vi "Main_Old.vi"() -> ()   [LabVIEW 2018]
uses:
  classes/Tushars Events Toolkit/Software/Modules/EventClient_ObjectReference.ctl
  classes/Variable Manager/VariableManager_Bool.vi
  Strict Type Controls/Settings Operation.ctl
  classes/Variable Manager/VariableManager_Double.vi
  <vilib>/Utility/file.llb/Write To Spreadsheet File (string).vi
panel:
  out "Quit":bool
  out "error out":errorcluster
  in  "error in (no error)":errorcluster
  in  "abort":bool
  in  "start":bool
  out "Test Status":bool
  out "statusMerlin":bool
  out "statusMC":bool
  out "statusPS":bool
  out "statusSM":bool
  in  "Start Merlin":bool
  in  "Start Monochromator":bool
  in  "Start Power Supply":bool
  in  "Start Source Meter":bool
  out "Value":dbl format="%#.7f mV"
  out "Measuring":dbl format="%#.7f nm"
  out "Voltage":dbl format="%#.7f mV"
  in  "tab":T1(tab)
  in  "Path For VT":path
  in  "exportVT":bool
  out "VTGraph":cluster{dbl[], dbl[]}(graph)
  in  "Test Mode":enum16{"Time Mode", "dV/dt Mode"}(ring)
  in  "Log Interval":u32=50 min=100 step=1 format="%.0f mSec"
  in  "Test Time":dbl step=1.0 format="%<%H:%M:%S>t"
  out "Time Remaining":dbl format="%<%H:%M:%S>t"
  in  "Target dV/dt":dbl format="%#.9f mV"
  in  "Lock In time":dbl step=1.0 format="%<%H:%M:%S>t"
  out "dV/dt":dbl format="%#.11f mV"
  out "Locked Time":dbl step=1.0 format="%<%H:%M:%S>t"
  in  "Perform Test After":T1(ring)=enum."Voltage Vs Wavelength"
  out "gratSetup?":bool
  in  "portD":bool
  in  "portA":bool
  in  "Path For Sweep":path
  in  "exportSweep":bool
  out "sweep":cluster{dbl[], dbl[]}[](graph)
  in  "Settling Time (ms)":dbl=5000.0
  in  "To":dbl=1000.0
  in  "Step":dbl=100.0
  in  "From":dbl=100.0
  in  "SetSlit":bool
  in  "SetGrating":bool
  in  "SetMonochromator":bool
  in  "Wavelength":dbl
  in  "Slit":string(combo)
  in  "GratingNo":u8=1 min=1 max=3 step=1
  in  "set Lock in":bool
  in  "#Stages":enum16{"None", "1 Pole", "2 Pole"}(ring)
  in  "Phase":enum16{"1 Phase", "2 Phase"}(ring)
  in  "SyncMode":T2(ring)
  in  "Time Const":T3(ring)
  in  "Sweep Results":i32(listbox)
  out "DCCurrent":dbl format="%#.4f A"
  out "DCVoltage":dbl format="%#.4f V"
  in  "Command":T4(ring)
  in  "Parm 4":dbl format="%#.6f"
  in  "Parm 3":dbl format="%#.6f"
  in  "openScript":bool
  in  "exportScript":bool
  in  "Path For Script":path
  in  "update":bool
  out "scriptGraph":cluster{dbl[], dbl[]}(graph)
  in  "Parm 2":dbl format="%#.6f"
  in  "Parm 1":dbl format="%#.6f"
  in  "script":i32(listbox)
  in  "add":bool
  in  "remove":bool
  in  "exportScriptResults":bool
  in  "Path For Script Results":path
  in  "Script Avg Interval":u32=50 min=100 step=1 format="%.0f mSec"
  # "Status"
  # "Test Type"
  # "Test Time"
  # "Voltage Results"
  # "Monochromator"
  # "Lock In Amplifier"
  # "Sweep"
  # "Merlin"
  # "NOTE:\n1. if this LED is OFF then GPIB is not connected...\n2. Close program before power off Instruments..."
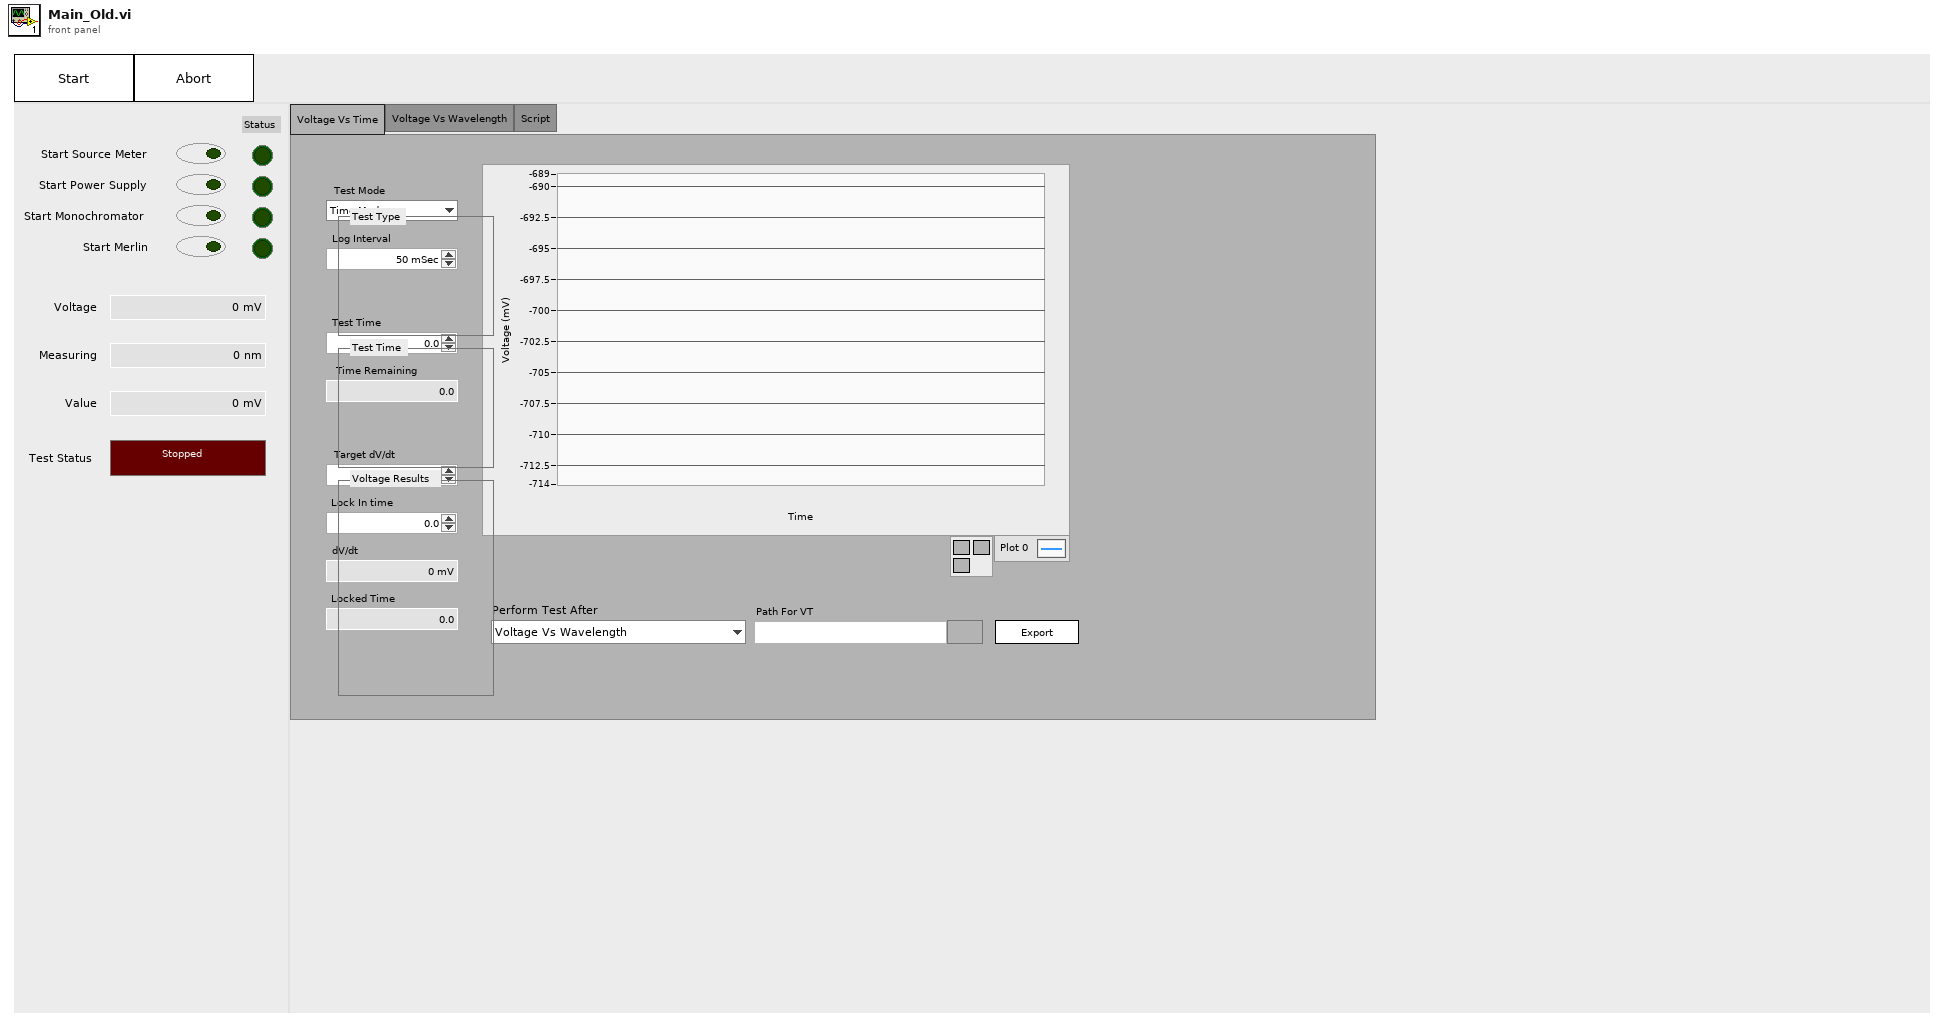
[diagram p1: front panel]
types:
  T1 = enum32{"Voltage Vs Time", "Voltage Vs Wavelength", "Script"}
  T2 = enum16{"Int Chop Off", "Int Chop On", "Ext Chop Off", "Ext Chop On"}
  T3 = enum16{".003s", ".010s", ".030s", ".100s", ".300s", "1.00s", "3.00s", "10.0s", "30.0s", "100s"}
  T4 = enum16{"selectChannel", "setDCVoltage", "setDCCurrent", "setVoltageSteps", "wait"}
  T5 = cluster{"startTime":u32, "lastUpdate":u32, "lastVoltage":dbl, "run?":bool, "From":dbl, "time":dbl[], "MerlinVal":dbl[], "SMVolt":dbl[], "sweepType":enum16{"ASC", "DESC"}, "Wavlnth":dbl[], "Test Mode":enum16{"Time Mode", "dV/dt Mode"}, "tab":enum32{"Voltage Vs Time", "Voltage Vs Wavelength", "Script"}, "script":string[][], "dV/dt":dbl[], "graphUpdate":u32}
  T6 = typedef "EventClient_ObjectReference.ctl" = refnum<k1>
  T7 = typedef "Settings Operation.ctl" = enum8{"Get Value", "Set Value", "Read File", "Write File", "Write Stored Value"}
  T8 = cluster{"GratingNo":u8, "Slit":string, "wavelength":dbl}
  T9 = cluster{"#Stages":enum16{"None", "1 Pole", "2 Pole"}, "Phase":enum16{"1 Phase", "2 Phase"}, "SyncMode":enum16{"Int Chop Off", "Int Chop On", "Ext Chop Off", "Ext Chop On"}, "Time Const":enum16{".003s", ".010s", ".030s", ".100s", ".300s", "1.00s", "3.00s", "10.0s", "30.0s", "100s"}}
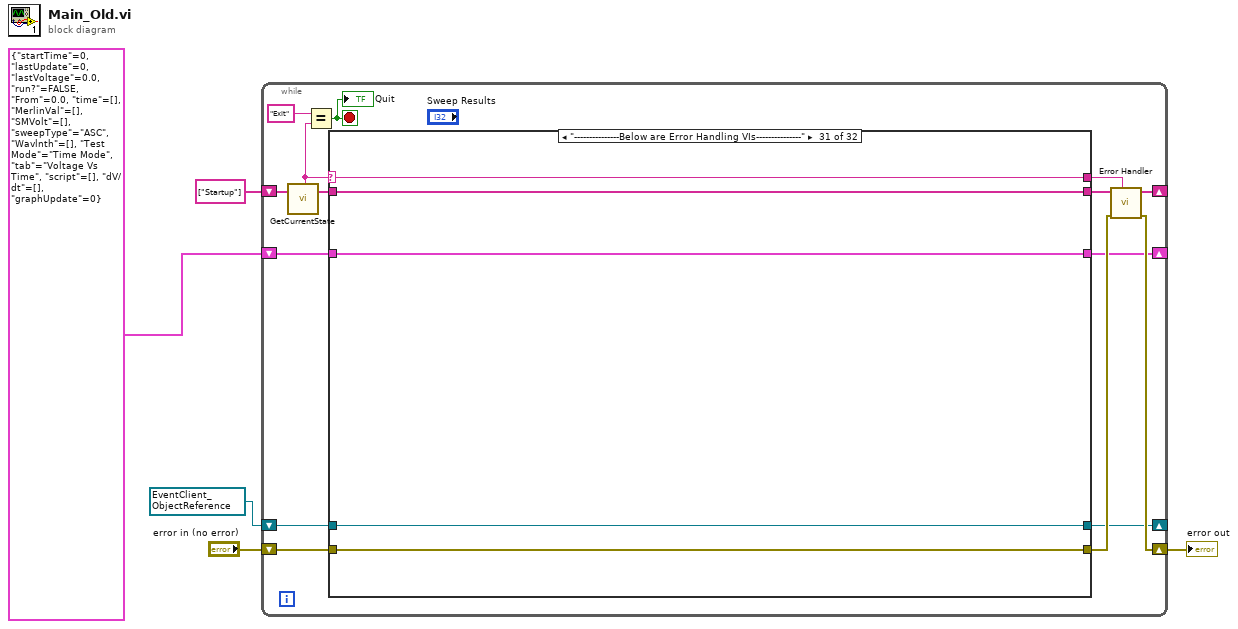
[diagram p0: block diagram]
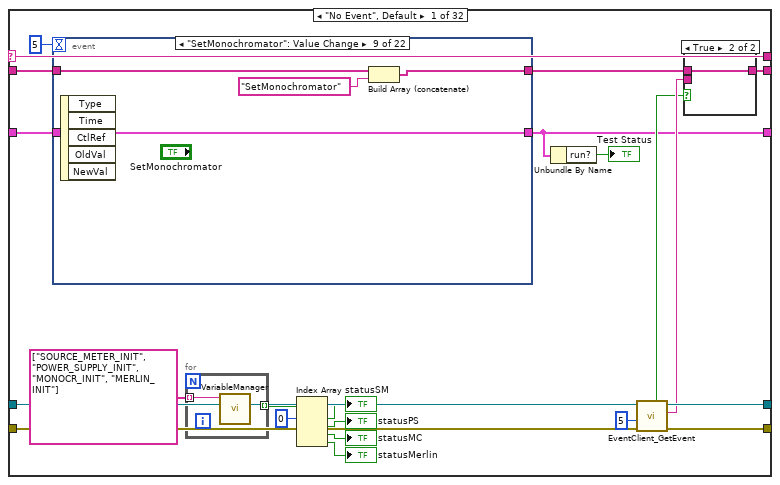
[diagram p2: hidden frame]
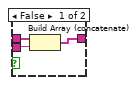
[diagram p3: hidden frame]
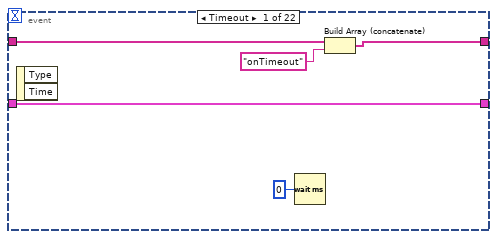
[diagram p4: hidden frame]
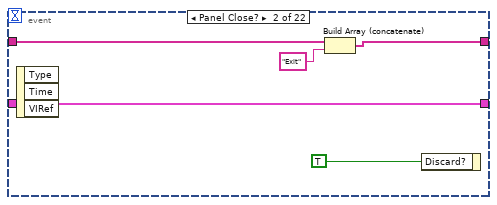
[diagram p5: hidden frame]
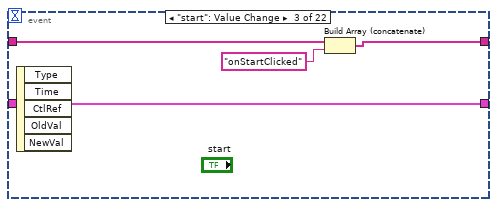
[diagram p6: hidden frame]
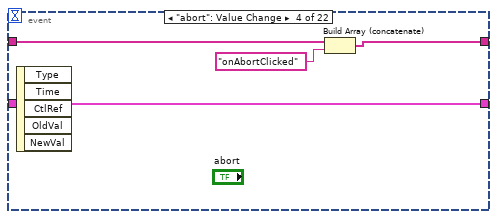
[diagram p7: hidden frame]
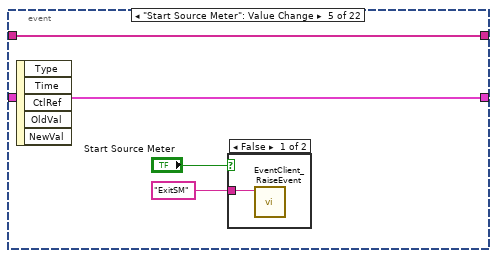
[diagram p8: hidden frame]
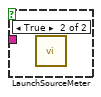
[diagram p9: hidden frame]
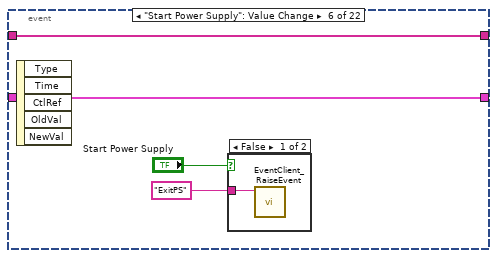
[diagram p10: hidden frame]
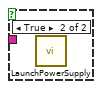
[diagram p11: hidden frame]
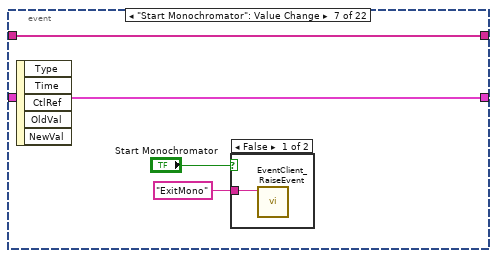
[diagram p12: hidden frame]
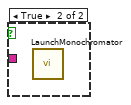
[diagram p13: hidden frame]
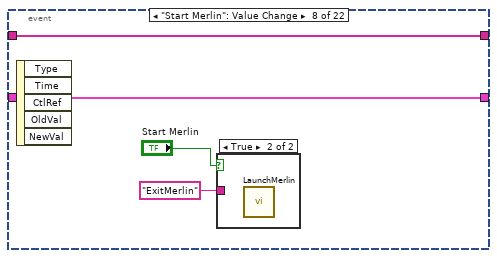
[diagram p14: hidden frame]
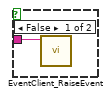
[diagram p15: hidden frame]
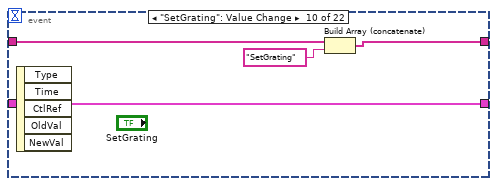
[diagram p16: hidden frame]
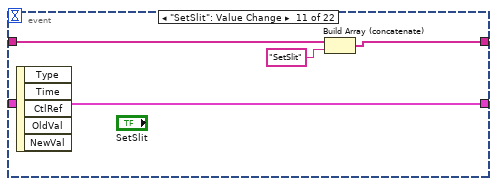
[diagram p17: hidden frame]
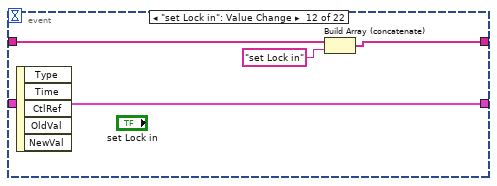
[diagram p18: hidden frame]
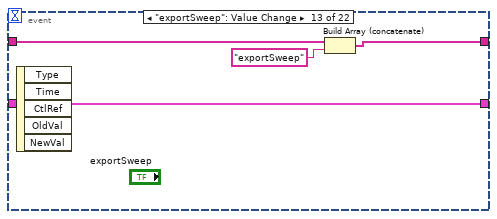
[diagram p19: hidden frame]
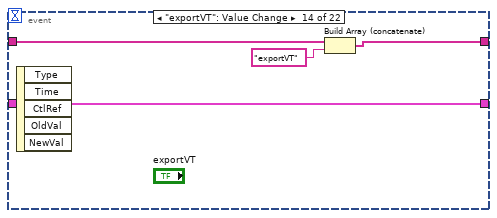
[diagram p20: hidden frame]
diagram:
  w2 = T6 refnum items=["EventClient"] ("reference")
  n1 = while {
    shift-right: [w16] -> _
    shift-left: string[] ["Startup"] ("State Array Out") -> [w20]
    shift-right: [w12] -> w3
    shift-left: "error in (no error)" -> [w13]
    shift-right: [w9] -> _
    shift-left: w2 -> [w8]
    shift-right: [w6] -> _
    shift-left: T5 {"startTime"=0, "lastUpdate"=0, "lastVoltage"=0.0, "run?"=FALSE, "From"=0.0, "time"=[], "MerlinVal"=[], "SMVolt"=[], "sweepType"=enum."ASC", "Wavlnth"=[], "Test Mode"=enum."Time Mode", "tab"=enum."Voltage Vs Time", "script"=[], "dV/dt"=[], "graphUpdate"=0} -> [w7]
    stop <- w17 stop-if-true
    n2 = call "GetCurrentState.vi"("State Array In"=w20) -> ("Current State"=w10:string, "State Array Out"=w19:string[])  [unwired: 17 in]
    n3 = Equal?(x="Exit", y=w10) -> (x = y?=w17:bool)
    "Quit" <- w17
    n4 = case shown="\"---------------Below are Error Handling VIs---------------\"" w10 {
      selector: w10 -> [w42 w172 w174 w184 w198 w208 w225 w242 w250 w258 w266 w290 w305 w315 w330 w348 w356 w367 w374 w386 w394 w404 w415 w420 w456 w496 w553 w577 w591 w655 w678 w694]
      tunnel: w19 -> [w41 w171 w180 w185 w199 w209 w226 w243 w251 w259 w267 w291 w306 w316 w331 w349 w364 w371 w378 w390 w395 w405 w416 w421 w457 w484 w554 w578 w582 w656 w677 w681]
      tunnel: [w32 w170 w180 w185 w199 w209 w226 w243 w251 w259 w267 w291 w306 w316 w331 w349 w364 w371 w378 w390 w395 w405 w416 w421 w457 w483 w554 w578 w583 w656 w677 w681] -> w15
      tunnel: [w37 w164 w175 w183 w197 w207 w224 w241 w249 w252 w260 w289 w304 w314 w329 w347 w357 w368 w375 w387 w393 w400 w411 w419 w450 w495 w552 w576 w590 w631 w676 errorcluster {"status"=FALSE, "code"=0, "source"=""} ("error in (no error)")] -> w11
      tunnel: [w42 w172 w174 w184 w198 w208 w225 w242 w250 w258 w266 w290 w305 w315 w330 w348 w356 w367 w374 w386 w394 w404 w415 w420 w456 w496 w553 w577 w591 w655 w678 w694] -> w14
      tunnel: w13 -> [w38 w159 w178 w183 w197 w207 w224 w241 w249 w253 w261 w289 w304 w314 w329 w347 w358 w369 w376 w388 w393 w402 w413 w419 w451 w495 w552 w576 w590 w632 w676 w682]
      tunnel: [w36 w162 w177 w182 w196 w206 w223 w240 w248 w257 w265 w288 w303 w313 w328 w346 w363 w370 w377 w389 w392 w398 w409 w418 w455 w494 w551 w575 w589 w654 w675 w680] -> w9
      tunnel: w8 -> [w39 _ w179 w182 w196 w206 w223 w240 w248 w257 w265 w288 w303 w313 w328 w346 w363 w370 w377 w389 w392 w403 w414 w418 w455 w494 w551 w575 w589 w654 w675 w680]
      tunnel: w7 -> [w23 w158 w173 w181 w195 w205 w222 w239 w247 w256 w264 w287 w302 w312 w327 w345 w355 w365 w372 w379 w391 w396 w408 w417 w426 w492 w539 w565 w588 w650 w674 w679]
      tunnel: [w22 w158 w173 w181 w195 w205 w222 w239 w247 w256 w264 w286 w301 w312 w327 w345 w355 w365 w372 w379 w391 w396 w408 w417 w453 w487 w538 w560 w588 w621 w674 w679] -> w6
      frame "No Event", Default {
        n5 = event shown="[8] \"SetMonochromator\": Value Change" {
          selector: _ -> [_ _ _ _ _ _ _ _ _ _ _ _ _ _ _ _ _ _ _ _ _ _]
          dyn-events: _ -> [_ _ _ _ _ _ _ _ _ _ _ _ _ _ _ _ _ _ _ _ _ _]
          timeout: 5 -> [_ _ _ _ _ _ _ _ _ _ _ _ _ _ _ _ _ _ _ _ _ _]
          tunnel: [w51 w56 w61 w65 w70 w75 w80 w85 w89 w93 w97 w101 w105 w109 w113 w117 w121 w125 w129 w133 w137 w141] -> w33
          tunnel: w41 -> [w53 w58 w62 w66 w70 w75 w80 w85 w90 w94 w98 w102 w106 w110 w114 w118 w122 w126 w130 w134 w138 w142]
          tunnel: w23 -> [w52 w54 w59 w63 w69 w74 w79 w84 w87 w91 w95 w99 w103 w107 w111 w115 w119 w123 w127 w131 w135 w139]
          tunnel: [w52 w54 w59 w63 w69 w74 w79 w84 w87 w91 w95 w99 w103 w107 w111 w115 w119 w123 w127 w131 w135 w139] -> w22
          event Timeout {
            n6 = event-data() -> ()  [unwired: 1 in, 2 out]
            n7 = Wait (ms)(milliseconds to wait=u32 0) -> ()  [unwired: 1 out]
            n8 = Build Array (concatenate)(w53, "onTimeout" ("x")) -> (w51:string[])
          }
          event Panel Close? {
            n9 = event-data() -> ()  [unwired: 1 in, 3 out]
            n10 = Build Array (concatenate)(w58, "Exit" ("x")) -> (w56:string[])
            n11 = event-data("Discard?"=TRUE) -> ()  [unwired: 1 in, 1 out]
          }
          event "start": Value Change {
            n12 = event-data() -> ()  [unwired: 1 in, 5 out]
            n13 = Build Array (concatenate)(w62, "onStartClicked" ("x")) -> (w61:string[])
          }
          event "abort": Value Change {
            n14 = event-data() -> ()  [unwired: 1 in, 5 out]
            n15 = Build Array (concatenate)(w66, "onAbortClicked" ("x")) -> (w65:string[])
          }
          event "Start Source Meter": Value Change {
            n16 = event-data() -> ()  [unwired: 1 in, 5 out]
            n17 = case shown="False" "Start Source Meter" {
              tunnel: "ExitSM" -> [w71 _]
              frame False {
                n18 = call "EventClient_RaiseEvent.vi"("Event"=w71) -> ()  [unwired: 10 in, 1 out]
              }
              frame True {
                n19 = call "LaunchSourceMeter.vi"() -> ()  [unwired: 11 in, 1 out]
              }
            }
          }
          event "Start Power Supply": Value Change {
            n20 = event-data() -> ()  [unwired: 1 in, 5 out]
            n21 = case shown="False" "Start Power Supply" {
              tunnel: "ExitPS" -> [w76 _]
              frame False {
                n22 = call "EventClient_RaiseEvent.vi"("Event"=w76) -> ()  [unwired: 10 in, 1 out]
              }
              frame True {
                n23 = call "LaunchPowerSupply.vi"() -> ()  [unwired: 11 in, 1 out]
              }
            }
          }
          event "Start Monochromator": Value Change {
            n24 = event-data() -> ()  [unwired: 1 in, 5 out]
            n25 = case shown="False" "Start Monochromator" {
              tunnel: "ExitMono" -> [w81 _]
              frame False {
                n26 = call "EventClient_RaiseEvent.vi"("Event"=w81) -> ()  [unwired: 10 in, 1 out]
              }
              frame True {
                n27 = call "LaunchMonochromator.vi"() -> ()  [unwired: 11 in, 1 out]
              }
            }
          }
          event "Start Merlin": Value Change {
            n28 = event-data() -> ()  [unwired: 1 in, 5 out]
            n29 = case shown="True" "Start Merlin" {
              tunnel: "ExitMerlin" -> [w86 _]
              frame False {
                n30 = call "EventClient_RaiseEvent.vi"("Event"=w86) -> ()  [unwired: 10 in, 1 out]
              }
              frame True {
                n31 = call "LaunchMerlin.vi"() -> ()  [unwired: 11 in, 1 out]
              }
            }
          }
          event "SetMonochromator": Value Change {
            n32 = event-data() -> ()  [unwired: 1 in, 5 out]
            n33 = Build Array (concatenate)(w90, "SetMonochromator" ("x")) -> (w89:string[])
          }
          event "SetGrating": Value Change {
            n34 = event-data() -> ()  [unwired: 1 in, 5 out]
            n35 = Build Array (concatenate)(w94, "SetGrating" ("x")) -> (w93:string[])
          }
          event "SetSlit": Value Change {
            n36 = event-data() -> ()  [unwired: 1 in, 5 out]
            n37 = Build Array (concatenate)(w98, "SetSlit" ("x")) -> (w97:string[])
          }
          event "set Lock in": Value Change {
            n38 = event-data() -> ()  [unwired: 1 in, 5 out]
            n39 = Build Array (concatenate)(w102, "set Lock in" ("x")) -> (w101:string[])
          }
          event "exportSweep": Value Change {
            n40 = event-data() -> ()  [unwired: 1 in, 5 out]
            n41 = Build Array (concatenate)(w106, "exportSweep" ("x")) -> (w105:string[])
          }
          event "exportVT": Value Change {
            n42 = event-data() -> ()  [unwired: 1 in, 5 out]
            n43 = Build Array (concatenate)(w110, "exportVT" ("x")) -> (w109:string[])
          }
          event "portA": Value Change {
            n44 = event-data() -> ()  [unwired: 1 in, 5 out]
            n45 = Build Array (concatenate)(w114, "portA" ("x")) -> (w113:string[])
          }
          event "portD": Value Change {
            n46 = event-data() -> ()  [unwired: 1 in, 5 out]
            n47 = Build Array (concatenate)(w118, "portD" ("x")) -> (w117:string[])
          }
          event "add": Value Change {
            n48 = event-data() -> ()  [unwired: 1 in, 5 out]
            n49 = Build Array (concatenate)(w122, "addStep" ("x")) -> (w121:string[])
          }
          event "remove": Value Change {
            n50 = event-data() -> ()  [unwired: 1 in, 5 out]
            n51 = Build Array (concatenate)(w126, "removeStep" ("x")) -> (w125:string[])
          }
          event "update": Value Change {
            n52 = event-data() -> ()  [unwired: 1 in, 5 out]
            n53 = Build Array (concatenate)(w130, "updateStep" ("x")) -> (w129:string[])
          }
          event "exportScript": Value Change {
            n54 = event-data() -> ()  [unwired: 1 in, 5 out]
            n55 = Build Array (concatenate)(w134, "exportScript" ("x")) -> (w133:string[])
          }
          event "exportScriptResults": Value Change {
            n56 = event-data() -> ()  [unwired: 1 in, 5 out]
            n57 = Build Array (concatenate)(w138, "exportScriptResults" ("x")) -> (w137:string[])
          }
          event "openScript": Value Change {
            n58 = event-data() -> ()  [unwired: 1 in, 5 out]
            n59 = Build Array (concatenate)(w142, "openScript" ("x")) -> (w141:string[])
          }
        }
        n60 = for {
          tunnel: string[] ["SOURCE_METER_INIT", "POWER_SUPPLY_INIT", "MONOCR_INIT", "MERLIN_INIT"] ("State Array Out") -> [w44] mode=indexing
          tunnel: [w43] -> w29 mode=indexing
          n61 = call-poly "VariableManager.vi"("Tag"=w44) -> ("Value out"=w43:bool)  [unwired: 7 in, 3 out]
        }
        n62 = Index Array(array=w29, index #1=0 ("index")) -> (element #1=→"statusSM":bool, element #2=→"statusPS":bool, element #3=→"statusMC":bool, element #4=→"statusMerlin":bool)  [unwired: 3 in]
        n63 = Unbundle By Name(w22) -> ("run?"=→"Test Status":bool)
        n64 = call "EventClient_GetEvent.vi"("error in (no error)"=w38, "timeout in ms (-1)"=5, "reference"=w39) -> ("error out"=w37:errorcluster, "Name"=w35:string, "reference out"=w36:T6, "timed out?"=w34:bool)  [unwired: 4 in, 1 out]
        n65 = case shown="True" w34 {
          tunnel: w33 -> [w47 w48]
          tunnel: w35 -> [w46 _]
          tunnel: [w45 w48] -> w32
          frame False {
            n66 = Build Array (concatenate)(w47, w46) -> (w45:string[])
          }
          frame True {
          }
        }
      }
      frame "Startup" {
        w147 = string[] ["Command", "Param 1", "Param 2"]  # script
        w148 = TRUE ("Start Source Meter")
        w145 = cluster{dbl[], dbl[]} {[], []} ("VTGraph")
        # "If Multiple instnances of this VI are possible \nthen make sure that client created in each instance gets a different Name"
        n67 = call "MonochromatorOffsets.vi"("Operation"=Settings_Operation."Read File", "error in (no error)"=w159) -> ("error out"=w152:errorcluster)  [unwired: 6 in, 3 out]
        n68 = call "LaunchPowerSupply.vi"("error in (no error)"=w152) -> ("error out"=w149:errorcluster)  [unwired: 10 in]
        n69 = local write "Log Interval"(u32 200 ("Log Interval")) -> ()
        n70 = local write "Target dV/dt"(1.0 ("Target dV/dt")) -> ()
        n71 = local write "Lock In time"(30.0 ("Lock In time")) -> ()
        n72 = local write "sweep"(cluster{dbl[], dbl[]}[] [] ("sweep")) -> ()
        n73 = local write "Test Time"(90.0 ("Locked Time")) -> ()
        n74 = local write "VTGraph"(w145) -> ()
        n75 = local write "scriptGraph"(w145) -> ()
        n76 = call "LaunchSourceMeter.vi"("error in (no error)"=w149) -> ("error out"=w150:errorcluster)  [unwired: 10 in]
        n77 = call "LaunchMerlin.vi"("error in (no error)"=w150) -> ("error out"=w144:errorcluster)  [unwired: 10 in]
        n78 = local write "tab"(T1."Voltage Vs Wavelength" ("tab")) -> ()
        n79 = call "LaunchMonochromator.vi"("error in (no error)"=w144) -> ("error out"=w151:errorcluster)  [unwired: 10 in]
        n80 = property on="script" class="MCListbox (strict)"("ColHdrString"=w147, "ItemNames"=string[][] [] ("Item Names")) -> ()  [unwired: 2 in, 2 out]
        n81 = Build Array (concatenate)(w171, string[] [] ("State Array Out")) -> (w170:string[])
        n82 = Call Chain() -> (call chain=w168:string[])
        n83 = local write "Start Source Meter"(w148) -> ()
        n84 = local write "Start Power Supply"(w148) -> ()
        n85 = local write "Start Monochromator"(w148) -> ()
        n86 = local write "Start Merlin"(w148) -> ()
        n87 = Index Array(array=w168, index=0) -> (element=w166:string)
        n88 = call "EventClient_Create.vi"("error in (no error)"=w151, "Instance Name"=w166) -> ("error out"=w165:errorcluster, "reference"=w163:T6)  [unwired: 8 in]
        n89 = call "EventClient_SubscribeEvents.vi"("error in (no error)"=w165, "Events"=string[] ["currGrating"], "reference"=w163) -> ("error out"=w164:errorcluster, "reference out"=w162:T6)  [unwired: 7 in]
      }
      frame "Exit" {
        w177 = T6 refnum items=["EventClient"] ("reference out")
        n90 = call "EventClient_Destroy.vi"("error in (no error)"=w178, "reference"=w179) -> ("error out"=w176:errorcluster)  [unwired: 9 in]
        n91 = call "EventClient_RaiseEvent.vi"("error in (no error)"=w176, "Event"=w174) -> ("error out"=w175:errorcluster)  [unwired: 9 in]
      }
      frame "---------------Below are UI Events---------------" {
        # "This State will never Execute\nIt is added just for improving code readability please do not remove this case"
      }
      frame "openScript" {
        w190 = string[][] []  # script
        n92 = Read from Text File() -> (text=w193:string, error out=w186:errorcluster)  [unwired: 4 in, 2 out]
        n93 = Spreadsheet String To Array(delimiter (Tab)=",", format string="%s", spreadsheet string=w193, array type (2D Dbl)=w190) -> (array=w189:string[][])
        n94 = call <vilib>:"Clear Errors.vi"("error in (no error)"=w186) -> ()  [unwired: 5 in, 2 out]
        n95 = Delete From Array(array=w189, index (row)=0) -> (deleted portion=w187:string[], array with subset deleted=w188:string[][])  [unwired: 2 in]
        n96 = property on="script" class="MCListbox (strict)"("ItemNames"=w188, "ColHdrString"=w187) -> ()  [unwired: 2 in, 2 out]
      }
      frame "exportScript" {
        n97 = property on="script" class="MCListbox (strict)"() -> ("ColHdrString"=w202:string[], "ItemNames"=w201:string[][])  [unwired: 2 in, 2 out]
        n98 = Build Array (concatenate)(w202, w201) -> (w204:string[][])
        n99 = call-poly <vilib>:"Write To Spreadsheet File.vi"("delimiter (\\t)"="," ("delimiter (\\t)"), "2D data"=w204, "file path (dialog if empty)"="Path For Script") -> ()  [unwired: 5 in, 1 out]
      }
      frame "updateStep" {
        n100 = local read "Command"() -> (w215:T4)
        n101 = local read "Parm 1"() -> (w214:dbl)
        n102 = local read "Parm 2"() -> (w213:dbl)
        n103 = local read "Parm 3"() -> (w211:dbl)
        n104 = local read "Parm 4"() -> (w210:dbl)
        n105 = Format Into String(w215) -> (resulting string=w217:string)  [unwired: 3 in, 1 out]
        n106 = Build Array(w214, w213, w211, w210) -> (w218:dbl[])
        n107 = property on="script" class="MCListbox (strict)"() -> ("ItemNames"=w221:string[][], "Value"=w219:i32)  [unwired: 2 in, 2 out]
        n108 = Number To Fractional String(number=w218) -> (F-format string=w216:string[])  [unwired: 3 in]
        n109 = Build Array (concatenate)(w217, w216) -> (w212:string[])
        n110 = Replace Array Subset(array=w221, new element=w212, index (row)=w219) -> (w220:string[][])  [unwired: 1 in]
        n111 = property on="script" class="MCListbox (strict)"("ItemNames"=w220) -> ()  [unwired: 2 in, 2 out]
      }
      frame "addStep" {
        n112 = property on="script" class="MCListbox (strict)"() -> ("ItemNames"=w236:string[][])  [unwired: 2 in, 2 out]
        n113 = Format Into String("Command") -> (resulting string=w232:string)  [unwired: 3 in, 1 out]
        n114 = Build Array("Parm 1", "Parm 2", "Parm 3", "Parm 4") -> (w233:dbl[])
        n115 = Number To Fractional String(number=w233, width (-)=i16 3 ("precision (6)")) -> (F-format string=w231:string[])  [unwired: 2 in]
        n116 = Build Array (concatenate)(w232, w231) -> (w230:string[])
        n117 = Build Array (concatenate)(w236, w230) -> (w235:string[][])
        n118 = property on="script" class="MCListbox (strict)"("ItemNames"=w235) -> ()  [unwired: 2 in, 2 out]
      }
      frame "removeStep" {
        n119 = property on="script" class="MCListbox (strict)"() -> ("ItemNames"=w246:string[][], "Value"=w244:i32)  [unwired: 2 in, 2 out]
        n120 = Delete From Array(array=w246, index (row)=w244) -> (array with subset deleted=w245:string[][])  [unwired: 2 in, 1 out]
        n121 = property on="script" class="MCListbox (strict)"("ItemNames"=w245) -> ()  [unwired: 2 in, 2 out]
      }
      frame "portA" {
        n122 = call "EventClient_RaiseEvent.vi"("error in (no error)"=w253, "Data"="!PORTIN A" ("concatenated string"), "Event"="MerlinWrite") -> ("error out"=w252:errorcluster)  [unwired: 8 in]
      }
      frame "portD" {
        n123 = call "EventClient_RaiseEvent.vi"("error in (no error)"=w261, "Data"="!PORTIN D" ("concatenated string"), "Event"="MerlinWrite") -> ("error out"=w260:errorcluster)  [unwired: 8 in]
      }
      frame "onStartClicked" {
        w275 = dbl[] [] ("time")
        n124 = local read "tab"() -> (w270:T1)
        n125 = local write "Locked Time"(0.0 ("Locked Time")) -> ()
        n126 = case shown="\"Voltage Vs Wavelength\"" w270 {
          tunnel: [0 0 2000] -> w268
          frame "Voltage Vs Time", Default {
            n127 = local write "VTGraph"(cluster{dbl[], dbl[]} {[], []} ("VTGraph")) -> ()
          }
          frame "Script" {
            n128 = local write "scriptGraph"(cluster{dbl[], dbl[]} {[], []} ("VTGraph")) -> ()
          }
          frame "Voltage Vs Wavelength" {
            n129 = local read "From"() -> (w297:dbl)
            n130 = property on="Sweep Results" class="MCListbox (strict)"("ItemNames"=string[][] [] ("Item Names")) -> ()  [unwired: 2 in, 2 out]
            n131 = local write "sweep"(cluster{dbl[], dbl[]}[] [] ("sweep")) -> ()
            n132 = call "setWavelenght.vi"("wavelength"=w297) -> ()  [unwired: 10 in, 1 out]
          }
        }
        n133 = Wait (ms)(milliseconds to wait=w268) -> ()  [unwired: 1 out]
        n134 = property on="script" class="MCListbox (strict)"() -> ("ItemNames"=w271:string[][])  [unwired: 2 in, 2 out]
        n135 = Less Or Equal?(x="From", y="To") -> (x <= y?=w281:bool)
        n136 = Select(t=enum16{"ASC", "DESC"}."ASC" ("sweepType"), s=w281, f=enum16{"ASC", "DESC"}."DESC" ("sweepType")) -> (s? t:f=w279:enum16{"ASC", "DESC"})
        n137 = Tick Count (ms)() -> (millisecond timer value=w269:u32)
        n138 = call-poly "VariableManager.vi"("Tag"="SM_VOLTAGE" ("String")) -> ("Value out"=w283:dbl)  [unwired: 6 in, 4 out]
        n139 = Bundle By Name(cluster=w287, "graphUpdate"=w269, "startTime"=w269, "lastUpdate"=w269, "run?"=TRUE, "lastVoltage"=w283, "time"=w275, "SMVolt"=w275, "MerlinVal"=w275, "Wavlnth"=w275, "sweepType"=w279, "From"="From", "tab"="tab", "Test Mode"="Test Mode", "script"=w271) -> (w286:T5)
        "Time Remaining" <- "Test Time"
      }
      frame "onAbortClicked" {
        n140 = Bundle By Name(cluster=w302, "run?"=FALSE) -> (w301:T5)
      }
      frame "exportSweep" {
        n141 = property on="Sweep Results" class="MCListbox (strict)"() -> ("ColHdrString"=w310:string[], "ItemNames"=w311:string[][])  [unwired: 2 in, 2 out]
        n142 = Build Array (concatenate)(w310, w311) -> (w309:string[][])
        n143 = call-poly <vilib>:"Write To Spreadsheet File.vi"("delimiter (\\t)"="," ("delimiter (\\t)"), "2D data"=w309, "file path (dialog if empty)"="Path For Sweep") -> ()  [unwired: 5 in, 1 out]
      }
      frame "exportVT" {
        n144 = local read "VTGraph"() -> (w318:cluster{dbl[], dbl[]})
        n145 = Unbundle(w318) -> (w323:dbl[], w320:dbl[])
        n146 = for {
          tunnel: w323 -> [w332] mode=indexing
          tunnel: "%<%H:%M:%S>t" ("format string") -> [w334]
          tunnel: [w333] -> w322 mode=indexing
          n147 = Format Into String(format string=w334, w332) -> (resulting string=w333:string)  [unwired: 2 in, 1 out]
        }
        n148 = Number To Fractional String(number=w320) -> (F-format string=w321:string[])  [unwired: 3 in]
        n149 = Build Array(w322, w321) -> (w317:string[][])
        n150 = Transpose 2D Array(2D array=w317) -> (transposed array=w319:string[][])
        n151 = call-poly <vilib>:"Write To Spreadsheet File.vi"("delimiter (\\t)"="," ("delimiter (\\t)"), "2D data"=w319, "file path (dialog if empty)"="Path For VT") -> ()  [unwired: 5 in, 1 out]
      }
      frame "exportScriptResults" {
        n152 = local read "scriptGraph"() -> (w337:cluster{dbl[], dbl[]})
        n153 = Unbundle(w337) -> (w342:dbl[], w339:dbl[])
        n154 = for {
          tunnel: w342 -> [w350] mode=indexing
          tunnel: "%<%H:%M:%S>t" ("format string") -> [w352]
          tunnel: [w351] -> w341 mode=indexing
          n155 = Format Into String(format string=w352, w350) -> (resulting string=w351:string)  [unwired: 2 in, 1 out]
        }
        n156 = Number To Fractional String(number=w339) -> (F-format string=w340:string[])  [unwired: 3 in]
        n157 = Build Array(w341, w340) -> (w336:string[][])
        n158 = Transpose 2D Array(2D array=w336) -> (transposed array=w338:string[][])
        n159 = call-poly <vilib>:"Write To Spreadsheet File.vi"("delimiter (\\t)"="," ("delimiter (\\t)"), "2D data"=w338, "file path (dialog if empty)"="Path For Script Results") -> ()  [unwired: 5 in, 1 out]
      }
      frame "SetMonochromator" {
        (unwired) "SetMono" ("Event")
        n160 = local read "GratingNo"() -> (w360:u8)
        n161 = local read "Slit"() -> (w359:string)
        n162 = Bundle By Name(cluster=T8 {"GratingNo"=0, "Slit"="", "wavelength"=0.0}, "GratingNo"=w360, "Slit"=w359, "wavelength"="Wavelength") -> (w362:T8)
        n163 = call "EventClient_RaiseEvent.vi"("error in (no error)"=w358, "Data"=w362, "Event"="SetWavelength") -> ("error out"=w357:errorcluster)  [unwired: 8 in]
      }
      frame "SetGrating" {
        n164 = call "EventClient_RaiseEvent.vi"("error in (no error)"=w369, "Data"="GratingNo", "Event"=w367) -> ("error out"=w368:errorcluster)  [unwired: 8 in]
      }
      frame "SetSlit" {
        n165 = call "EventClient_RaiseEvent.vi"("error in (no error)"=w376, "Data"="Slit", "Event"=w374) -> ("error out"=w375:errorcluster)  [unwired: 8 in]
      }
      frame "set Lock in" {
        n166 = Bundle By Name(cluster=T9 {"#Stages"=enum."None", "Phase"=enum."1 Phase", "SyncMode"=enum."Int Chop Off", "Time Const"=enum.".003s"}, "#Stages"="#Stages", "Phase"="Phase", "SyncMode"="SyncMode", "Time Const"="Time Const") -> (w385:T9)
        n167 = call "EventClient_RaiseEvent.vi"("error in (no error)"=w388, "Data"=w385, "Event"=w386) -> ("error out"=w387:errorcluster)  [unwired: 8 in]
      }
      frame "---------------Below are Menu Events---------------" {
        # "This State will never Execute\nIt is added just for improving code readability please do not remove this case"
      }
      frame "---------------Below are Client Events---------------" {
        # "To Handle Event Duplicate this case. If Event Does not have any data then remove\nGet Event Data and variant to data VIs"
        # "Connect Proper DataType Here"
        n168 = call "EventClient_GetEventData.vi"("error in (no error)"=w402, "reference"=w403) -> ("error out"=w401:errorcluster, "Data"=w399:variant, "reference out"=w398:T6)  [unwired: 7 in]
        n169 = Variant To Data(error in=w401, type=variant, Variant=w399) -> (error out=w400:errorcluster)  [unwired: 1 out]
      }
      frame "currGrating" {
        n170 = call "EventClient_GetEventData.vi"("error in (no error)"=w413, "reference"=w414) -> ("error out"=w412:errorcluster, "Data"=w410:variant, "reference out"=w409:T6)  [unwired: 7 in]
        n171 = Variant To Data(error in=w412, type=u32 0, Variant=w410) -> (data=w406:u32, error out=w411:errorcluster)
        n172 = local write "GratingNo"(w406) -> ()
      }
      frame "---------------Below are Subroutine states---------------" {
      }
      frame "executeScript" {
        n173 = Unbundle By Name(w426) -> ("script"=w422:string[][], "lastUpdate"=w443:u32, "graphUpdate"=w436:u32)
        n174 = Unbundle By Name(w426) -> ("startTime"=w446:u32, "time"=w432:dbl[], "SMVolt"=w431:dbl[])
        n175 = Empty Array?(array=w422) -> (empty?=w423:bool)
        n176 = call "executeScript.vi"("script"=w422, "lastUpdate"=w443, "error in (no error)"=w451) -> ("scriptOut"=w454:string[][], "lastUpdate 2"=w437:u32, "error out"=w450:errorcluster)  [unwired: 5 in]
        n177 = Increment(x="script") -> (x+1=w445:i32)
        n178 = Tick Count (ms)() -> (millisecond timer value=w424:u32)
        n179 = Not(x=w423) -> (.not. x?=w452:bool)
        n180 = Subtract(x=w424, y=w446) -> (x-y=w448:u32)
        n181 = Subtract(x=w424, y=w436) -> (x-y=w435:u32)
        n182 = local write "script"(w445) -> ()
        n183 = Greater Or Equal?(x=w435, y="Script Avg Interval") -> (x >= y?=w433:bool)
        n184 = Divide(x=w448, y=u32 1000) -> (x/y=w429:dbl)
        n185 = call-poly "VariableManager.vi"("Tag"="SM_VOLTAGE") -> ("Value out"=w430:dbl)  [unwired: 6 in, 4 out]
        n186 = local write "Voltage"(w430) -> ()
        n187 = case shown="True" w433 {
          tunnel: w432 -> [w464 w470]
          tunnel: w431 -> [w463 w469]
          tunnel: w430 -> [w462 _]
          tunnel: w429 -> [w461 _]
          tunnel: [w460 w468] -> w428
          tunnel: [w459 w468] -> w427
          tunnel: w426 -> [w458 w467]
          tunnel: [w458 w466] -> w425
          tunnel: w424 -> [_ w465]
          frame False {
            n188 = Build Array (concatenate)(w464, w462) -> (w460:dbl[])
            n189 = Build Array (concatenate)(w463, w461) -> (w459:dbl[])
          }
          frame True {
            w468 = dbl[] []
            n190 = call "AvarageSamples.vi"("samples"=w470) -> ("Avg"=w471:dbl)  [unwired: 10 in]
            n191 = call "AvarageSamples.vi"("samples"=w469) -> ("Avg"=w472:dbl)  [unwired: 10 in]
            n192 = local read "scriptGraph"() -> (w477:cluster{dbl[], dbl[]})
            n193 = Unbundle(w477) -> (w476:dbl[], w473:dbl[])
            n194 = Build Array (concatenate)(w476, w471) -> (w475:dbl[])
            n195 = Build Array (concatenate)(w473, w472) -> (w474:dbl[])
            n196 = Bundle By Name(cluster=w467, "lastUpdate"=w465) -> (w466:T5)
            n197 = Bundle(cluster=w477, w475, w474) -> (→"scriptGraph":cluster{dbl[], dbl[]})
          }
        }
        n198 = for {
          tunnel: string[] ["DCVoltage", "DCCurrent"] ("State Array Out") -> [w480] mode=indexing
          tunnel: [w479] -> w441 mode=indexing
          n199 = call-poly "VariableManager.vi"("Tag"=w480) -> ("Value out"=w479:dbl)  [unwired: 6 in, 4 out]
        }
        n200 = Index Array(array=w441, index #1=0 ("index")) -> (element #1=w438:dbl, element #2=w439:dbl)  [unwired: 1 in]
        n201 = local write "DCVoltage"(w438) -> ()
        n202 = local write "DCCurrent"(w439) -> ()
        n203 = Bundle By Name(cluster=w425, "run?"=w452, "script"=w454, "time"=w428, "SMVolt"=w427, "lastUpdate"=w437) -> (w453:T5)
      }
      frame "checkForAbort" {
        n204 = Unbundle By Name(w492) -> ("lastVoltage"=w491:dbl, "Test Mode"=w493:enum16{"Time Mode", "dV/dt Mode"}, "tab"=w486:T1)
        n205 = local read "Voltage"() -> (w490:dbl)
        n206 = case shown="\"dV/dt Mode\"" w493 {
          tunnel: w492 -> [w502 w526]
          tunnel: [w502 w526] -> w488
          tunnel: [w498 w505] -> w485
          tunnel: w490 -> [w501 w519]
          tunnel: [w501 w519] -> w489
          tunnel: w491 -> [_ w516]
          tunnel: w486 -> [w500 w507]
          tunnel: [w500 w512] -> w482
          tunnel: w484 -> [w499 w509]
          tunnel: [w499 w510] -> w483
          tunnel: [w498 w505] -> w481
          frame "Time Mode", Default {
            n207 = local read "Time Remaining"() -> (w503:dbl)
            n208 = Greater Or Equal To 0?(x=w503) -> (x >= 0?=w498:bool)
          }
          frame "dV/dt Mode" {
            n209 = local read "Log Interval"() -> (w523:u32)
            n210 = local read "Locked Time"() -> (w513:dbl)
            n211 = Subtract(x=w519, y=w516) -> (x-y=w525:dbl)
            n212 = Divide(x=w523, y=u32 1000) -> (x/y=w522:dbl)
            n213 = Divide(x=w525, y=w522) -> (x/y=w527:dbl)
            n214 = Add(x=w522, y=w513) -> (x+y=w520:dbl)
            n215 = Absolute Value(x=w527) -> (abs(x)=w514:dbl)
            "dV/dt" <- w514
            n216 = Less Or Equal?(x=w514, y="Target dV/dt") -> (x <= y?=w521:bool)
            n217 = case shown="False" w521 {
              tunnel: [0.0 ("Locked Time") w534] -> w517
              tunnel: w520 -> [_ w534]
              frame False {
              }
              frame True {
              }
            }
            "Locked Time" <- w517
            n218 = Build Array (concatenate)(w509, "onStartClicked" ("String")) -> (w508:string[])
            n219 = Equal?(x=w507, y="Perform Test After") -> (x = y?=w504:bool)
            n220 = Greater Or Equal?(x="Lock In time", y=w517) -> (x >= y?=w505:bool)
            n221 = case shown="False" w505 {
              tunnel: [w531 w532] -> w510
              tunnel: w509 -> [w530 w532]
              tunnel: w508 -> [w529 _]
              tunnel: w504 -> [w528 _]
              frame False {
                n222 = Select(t=w530, s=w528, f=w529) -> (s? t:f=w531:string[])
              }
              frame True {
              }
            }
            n223 = Select(t=w507, s=w505, f="Perform Test After") -> (s? t:f=w512:T1)
          }
        }
        n224 = case shown="False" w481 {
          tunnel: w482 -> [w497 _]
          frame False {
            n225 = local write "tab"(w497) -> ()
          }
          frame True {
          }
        }
        n226 = Bundle By Name(cluster=w488, "lastVoltage"=w489, "run?"=w485, "tab"=w482) -> (w487:T5)
      }
      frame "accumValues" {
        n227 = Unbundle By Name(w539) -> ("startTime"=w547:u32, "time"=w542:dbl[], "SMVolt"=w541:dbl[], "Test Mode"=w535:enum16{"Time Mode", "dV/dt Mode"})
        n228 = local read "Test Time"() -> (w546:dbl)
        n229 = Tick Count (ms)() -> (millisecond timer value=w548:u32)
        n230 = Subtract(x=w548, y=w547) -> (x-y=w549:u32)
        n231 = Divide(x=w549, y=u32 1000) -> (x/y=w540:dbl)
        n232 = call-poly "VariableManager.vi"("Tag"="SM_VOLTAGE") -> ("Value out"=w543:dbl)  [unwired: 6 in, 4 out]
        n233 = Subtract(x=w546, y=w540) -> (x-y=w545:dbl)
        n234 = Build Array (concatenate)(w542, w540) -> (w537:dbl[])
        n235 = Build Array (concatenate)(w541, w543) -> (w536:dbl[])
        n236 = Array Size(array=w536) -> ()  [unwired: 1 out]
        n237 = Bundle By Name(cluster=w539, "time"=w537, "SMVolt"=w536) -> (w538:T5)
        n238 = case shown="\"dV/dt Mode\"" w535 {
          tunnel: w545 -> [w555 _]
          frame "Time Mode", Default {
            n239 = local write "Time Remaining"(w555) -> ()
          }
          frame "dV/dt Mode" {
            n240 = local write "Time Remaining"(0.0 ("Time Remaining")) -> ()
          }
        }
      }
      frame "updateGraph" {
        w559 = dbl[] [] ("time")
        n241 = Unbundle By Name(w565) -> ("time"=w566:dbl[], "SMVolt"=w564:dbl[], "lastVoltage"=w563:dbl)
        n242 = Array Size(array=w566) -> (size(s)=w574:i32)
        n243 = Decrement(x=w574) -> (x-1=w573:i32)
        n244 = Index Array(array=w566, index #1=w573, index #2=0 ("index")) -> (element #1=w567:dbl)  [unwired: 1 out]
        n245 = call "getAvarageVoltageForInterval.vi"("lastVal"=w563, "voltages"=w564, "timeArray"=w566) -> ("avarage"=w557:dbl)  [unwired: 8 in]
        n246 = local read "VTGraph"() -> (w561:cluster{dbl[], dbl[]})
        n247 = local write "Voltage"(w557) -> ()
        n248 = Unbundle(w561) -> (w572:dbl[], w571:dbl[])
        n249 = Build Array (concatenate)(w572, w567) -> (w570:dbl[])
        n250 = Build Array (concatenate)(w571, w557) -> (w569:dbl[])
        n251 = Tick Count (ms)() -> (millisecond timer value=w558:u32)
        n252 = Bundle(w570, w569) -> (→"VTGraph":cluster{dbl[], dbl[]})  [unwired: 1 in]
        n253 = Bundle By Name(cluster=w565, "time"=w559, "SMVolt"=w559, "lastUpdate"=w558) -> (w560:T5)
      }
      frame "onTimeout" {
        n254 = Unbundle By Name(w588) -> ("run?"=w587:bool, "tab"=w586:T1, "Test Mode"=w585:enum16{"Time Mode", "dV/dt Mode"}, "lastUpdate"=w584:u32)
        n255 = call-poly "VariableManager.vi"("Operation"=enum16{"Get Tag", "Set Tag"}."Get Tag", "Tag"="GratingChange?") -> ("Value out"=w579:bool)  [unwired: 6 in, 3 out]
        "gratSetup?" <- w579
        n256 = case shown="True" w587 {
          tunnel: w586 -> [_ w607]
          tunnel: w585 -> [_ _]
          tunnel: w584 -> [_ w606]
          tunnel: [w599 w604] -> w583
          tunnel: w582 -> [w599 w605]
          tunnel: w579 -> [_ w602]
          frame False {
            n257 = for {
              tunnel: string[] ["SM_VOLTAGE", "MERLIN_VALUE", "DCVoltage", "DCCurrent"] ("State Array Out") -> [w601] mode=indexing
              tunnel: [w600] -> w597 mode=indexing
              n258 = call-poly "VariableManager.vi"("Tag"=w601) -> ("Value out"=w600:dbl)  [unwired: 6 in, 4 out]
            }
            n259 = Index Array(array=w597, index #1=0 ("index")) -> (element #1=→"Voltage":dbl, element #2=→"Value":dbl, element #3=→"DCVoltage":dbl, element #4=→"DCCurrent":dbl)  [unwired: 3 in]
          }
          frame True {
            n260 = case shown="\"Voltage Vs Time\", Default" w607 {
              tunnel: [w609 w617 string[] ["executeScript"] ("State Array Out")] -> w603
              tunnel: w606 -> [w613 _ _]
              tunnel: w602 -> [_ w616 _]
              frame "Voltage Vs Time", Default {
                n261 = Tick Count (ms)() -> (millisecond timer value=w615:u32)
                n262 = Subtract(x=w615, y=w613) -> (x-y=w614:u32)
                n263 = Greater Or Equal?(x=w614, y="Log Interval") -> (x >= y?=w611:bool)
                n264 = Select(t=string[] ["updateGraph", "checkForAbort"] ("State Array Out"), s=w611, f=string[] ["accumValues"] ("State Array Out")) -> (s? t:f=w609:string[])
              }
              frame "Voltage Vs Wavelength" {
                n265 = Select(t=string[] [] ("State Array Out"), s=w616, f=string[] ["sweep"] ("State Array Out")) -> (s? t:f=w617:string[])
              }
              frame "Script" {
              }
            }
            n266 = Build Array (concatenate)(w605, w603) -> (w604:string[])
          }
        }
      }
      frame "sweep" {
        n267 = Unbundle By Name(w650) -> ("Wavlnth"=w653:dbl[], "MerlinVal"=w652:dbl[], "SMVolt"=w651:dbl[], "sweepType"=w643:enum16{"ASC", "DESC"}, "From"=w642:dbl)
        n268 = local read "To"() -> (w635:dbl)
        n269 = case shown="\"ASC\"" w643 {
          tunnel: w642 -> [w664 w669]
          tunnel: "Step" -> [w668 w673]
          tunnel: [w667 w672] -> w633
          tunnel: w635 -> [w666 w671]
          tunnel: [w665 w670] -> w622
          tunnel: [w664 w669] -> w625
          frame "DESC" {
            n270 = Subtract(x=w664, y=w668) -> (x-y=w667:dbl)
            n271 = Less Or Equal?(x=w666, y=w664) -> (x <= y?=w665:bool)
          }
          frame "ASC" {
            n272 = Add(x=w669, y=w673) -> (x+y=w672:dbl)
            n273 = Greater Or Equal?(x=w671, y=w669) -> (x >= y?=w670:bool)
          }
        }
        "Measuring" <- w625
        n274 = call "setWavelenght.vi"("error in (no error)"=w632, "wavelength"=w625) -> ("error out"=w634:errorcluster)  [unwired: 9 in]
        n275 = flat-sequence {
          tunnel: w634 -> [w663]
          tunnel: [w663] -> w638
          tunnel: "Settling Time (ms)" -> [w662]
          frame #0 {
            n276 = Wait (ms)(milliseconds to wait=w662) -> ()  [unwired: 1 out]
          }
        }
        n277 = for {
          tunnel: string[] ["SM_VOLTAGE", "MERLIN_VALUE"] ("State Array Out") -> [w661] mode=indexing
          shift-right: [w660] -> w631
          shift-left: w638 -> [w659]
          tunnel: [w658] -> w637 mode=indexing
          n278 = call-poly "VariableManager.vi"("error in (no error)"=w659, "Tag"=w661) -> ("error out"=w660:errorcluster, "Value out"=w658:dbl)  [unwired: 5 in, 3 out]
        }
        n279 = Index Array(array=w637, index #1=0 ("index")) -> (element #1=w623:dbl, element #2=w624:dbl)  [unwired: 1 in]
        n280 = Build Array(w625, w624, w623) -> (w627:dbl[])
        n281 = property on="Sweep Results" class="MCListbox (strict)"() -> ("ItemNames"=w630:string[][])  [unwired: 2 in, 2 out]
        n282 = local write "Voltage"(w623) -> ()
        n283 = Number To Fractional String(number=w627, width (-)=i16 8) -> (F-format string=w626:string[])  [unwired: 2 in]
        n284 = Build Array (concatenate)(w653, w625) -> (w646:dbl[])
        n285 = Build Array (concatenate)(w652, w624) -> (w645:dbl[])
        n286 = Build Array (concatenate)(w651, w623) -> (w644:dbl[])
        n287 = Build Array (concatenate)(w630, w626) -> (w629:string[][])
        n288 = Bundle(w646, w645) -> (w648:cluster{dbl[], dbl[]})  [unwired: 1 in]
        n289 = Bundle(w646, w644) -> (w649:cluster{dbl[], dbl[]})  [unwired: 1 in]
        n290 = property on="Sweep Results" class="MCListbox (strict)"("ItemNames"=w629) -> ()  [unwired: 2 in, 2 out]
        n291 = Bundle By Name(cluster=w650, "Wavlnth"=w646, "MerlinVal"=w645, "SMVolt"=w644, "run?"=w622, "From"=w633) -> (w621:T5)
        n292 = case shown="False" w622 {
          tunnel: w621 -> [_ _]
          frame False {
            n293 = local read "From"() -> (w657:dbl)
            n294 = call "setWavelenght.vi"("wavelength"=w657) -> ()  [unwired: 10 in, 1 out]
          }
          frame True {
          }
        }
        n295 = Build Array(w648, w649) -> (→"sweep":cluster{dbl[], dbl[]}[])
      }
      frame "---------------Below are Error Handling VIs---------------" {
      }
      frame "Error" {
        n296 = Call Chain() -> (call chain=w689:string[])
        n297 = for {
          tunnel: w689 -> [w697] mode=indexing
          shift-right: [w695] -> w686
          shift-left: "" -> [w698]
          n298 = Concatenate Strings(w698, w697, " -> ") -> (w695:string)
        }
        n299 = Unbundle By Name(w682) -> ("code"=w684:i32, "source"=w683:string)
        n300 = Match Pattern(string=w683, regular expression=":") -> (before substring=w687:string, after substring=w691:string)  [unwired: 1 in, 2 out]
        n301 = Format Into String(format string="Error Occured In\"%s\" state of \"%s\" VI\nError Code: %d\nError Description: \"%s\"", w687, w686, w684, w691) -> (resulting string=w690:string)  [unwired: 2 in, 1 out]
        n302 = One Button Dialog(message=w690) -> ()  [unwired: 1 in, 1 out]
      }
    }
    n303 = call "Error Handler.vi"("Current State"=w14, "error in (no error)"=w11, "Msg Queue In"=w15) -> ("error out"=w12:errorcluster, "Msg Queue Out"=w16:string[])  [unwired: 7 in]
  }
  "error out" <- w3
